vi "校准信息写入.vi"(8 "Error in":errorcluster caption="Error in (no error)", 10 "校准信息读取":T1 {"校准类型" items=["单点校准"=1, "两点校准"=2, "三点校准"=3]}, 11 "Slave ID":u8=1) -> (0 "error out":errorcluster)   [LabVIEW 2016, in "斯坦道原位多参数.lvlib"]
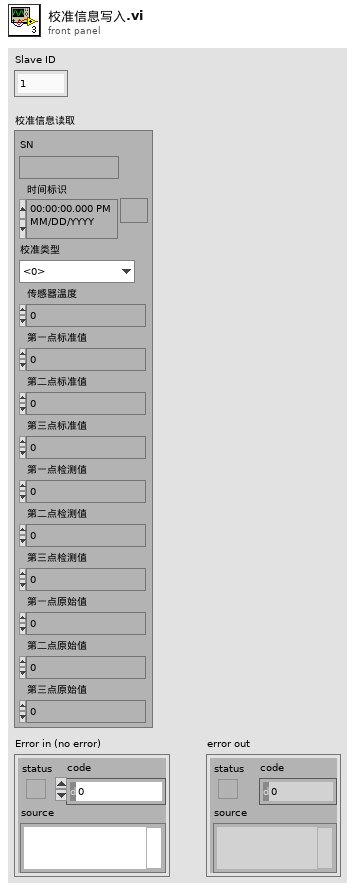
[diagram p1: front panel]
types:
  T1 = cluster{"SN":string, "时间标识":timestamp, "校准类型":u16, "传感器温度":sgl, "第一点标准值":sgl, "第二点标准值":sgl, "第三点标准值":sgl, "第一点检测值":sgl, "第二点检测值":sgl, "第三点检测值":sgl, "第一点原始值":sgl, "第二点原始值":sgl, "第三点原始值":sgl}
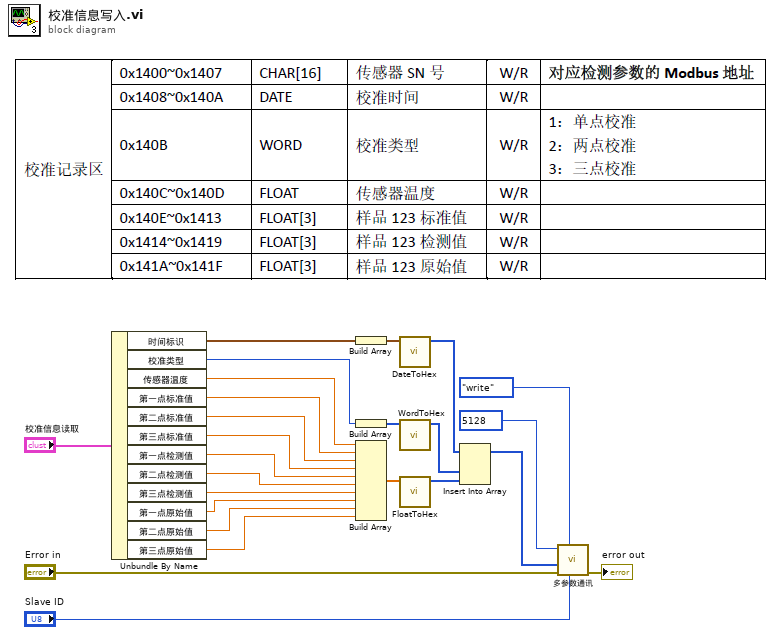
[diagram p0: block diagram]
diagram:
  n1 = Unbundle By Name("校准信息读取") -> ("时间标识"=w19:timestamp, "校准类型"=w17:u16, "传感器温度"=w15:sgl, "第一点标准值"=w14:sgl, "第二点标准值"=w13:sgl, "第三点标准值"=w12:sgl, "第一点检测值"=w11:sgl, "第二点检测值"=w10:sgl, "第三点检测值"=w9:sgl, "第一点原始值"=w8:sgl, "第二点原始值"=w7:sgl, "第三点原始值"=w6:sgl)
  n2 = Build Array(w19) -> (w18:timestamp[])
  n3 = Build Array(w17) -> (w16:u16[])
  n4 = Build Array(w15, w14, w13, w12, w11, w10, w9, w8, w7, w6) -> (w5:sgl[])
  n5 = call "DateToHex.vi"("DATE"=w18) -> ("数组"=w4:u16[])  [unwired: 10 in]
  n6 = call "WordToHex.vi"("WORD"=w16) -> ("数组"=w3:u16[])  [unwired: 10 in]
  n7 = call "FloatToHex.vi"("浮点数"=w5) -> ("DCBA整形输出"=w2:u16[])  [unwired: 10 in]
  n8 = Insert Into Array(array=w4, new element #1=w3, new element #2=w2) -> (w1:u16[])  [unwired: 1 in]
  n9 = call "多参数通讯.vi"("Slave ID"="Slave ID", "STEP"=enum16{"open", "read", "write", "close"}."write", "Error in"="Error in", "values"=w1, "starting address"=u16 5128) -> ("error out"=→"error out":errorcluster)  [unwired: 4 in, 2 out]
